vi "SetMotors (SubVI).vi"(6 "Oikea":dbl, 9 "Etu":dbl, 10 "Vasen":dbl, 11 "Taka":dbl) -> ()   [LabVIEW 2018]
uses:
  <vilib>/Utility/error.llb/Error Cluster From Error Code.vi
  <vilib>/myRIO/Common/Instrument Driver Framework/myRIO v1.0/PWM/vis/myRIO v1.0 Write PWM.vi
  <vilib>/myRIO/Instrument Drivers/Onboard IO/PWM/PWM.lvlib
panel:
  out "error out":errorcluster
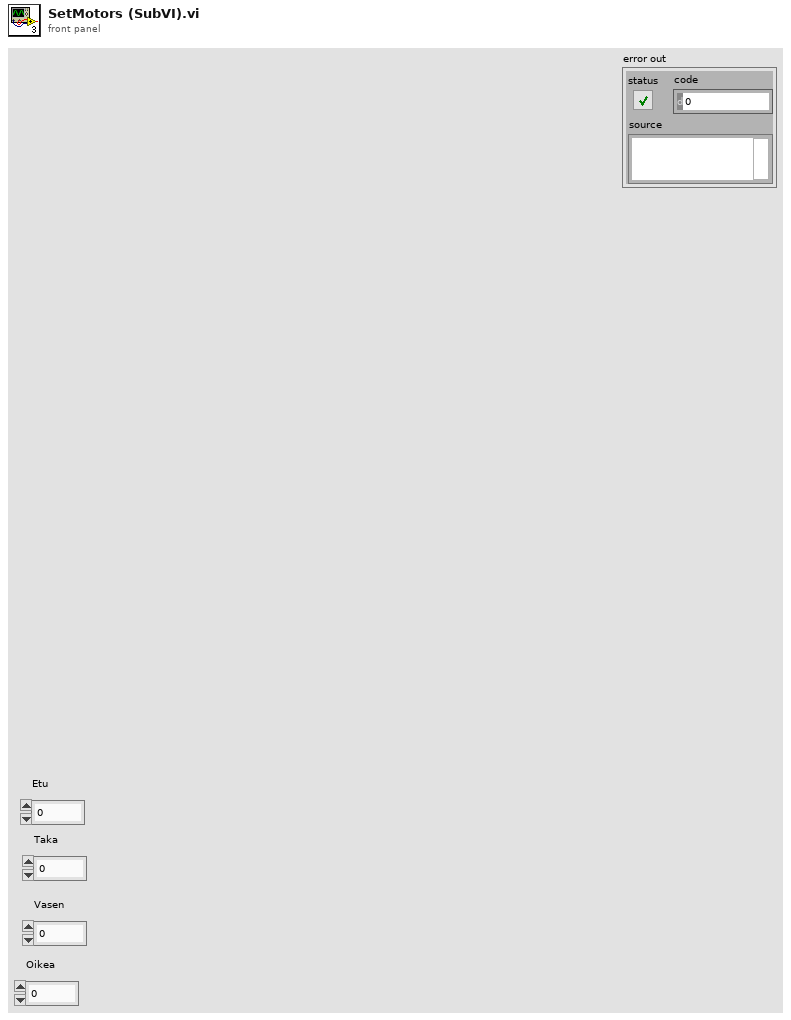
[diagram p1: front panel]
types:
  T1 = typedef "PWM.lvlib/PWM Reference.ctl" = cluster{"myRIO Reference":T2, "PWM Channels Enum":T6, "PWM Configuration":T7}
  T2 = typedef "myRIO Generic Hardware Reference.ctl" = cluster{"myRIO Model":T3, "myRIO Hardware Reference":T4}
  T3 = typedef "Hardware Version Enum.ctl" = enum16{"Unknown", "myRIO-1900", "myRIO-1950", "roboRIO", "NI ELVIS RIO CM", "ELVIS III"}
  T4 = typedef "myRIO v1.0 Reference.ctl" = cluster{"Generic FPGA Reference":T5, "Allow multiple opens":bool}
  T5 = typedef "Generic FPGA Reference.ctl" = refnum<k20>
  T6 = typedef "PWM Channels Enum.ctl" = enum16{"Not Connected", "C/PWM0", "C/PWM1", "A/PWM0", "A/PWM1", "A/PWM2", "A/PWM3", "A/PWM4", "A/PWM5", "A/PWM6", "A/PWM7", "A/PWM8", "A/PWM9", "A/PWM10", "A/PWM11", "A/PWM12", "A/PWM13", "A/PWM14", "A/PWM15", "A/PWM16", "A/PWM17", "A/PWM18", "A/PWM19", "B/PWM0", "B/PWM1", "B/PWM2", "B/PWM3", "B/PWM4", "B/PWM5", "B/PWM6", "B/PWM7", "B/PWM8", "B/PWM9", "B/PWM10", "B/PWM11", "B/PWM12", "B/PWM13", "B/PWM14", "B/PWM15", "B/PWM16", "B/PWM17", "B/PWM18", "B/PWM19", "PWM/PWM0", "PWM/PWM1", "PWM/PWM2", "PWM/PWM3", "PWM/PWM4", "PWM/PWM5", "PWM/PWM6", "PWM/PWM7", "PWM/PWM8", "PWM/PWM9"}
  T7 = typedef "PWM.lvlib/PWM Configuration.ctl" = cluster{"Frequency":dbl, "Duty Cycle":dbl}
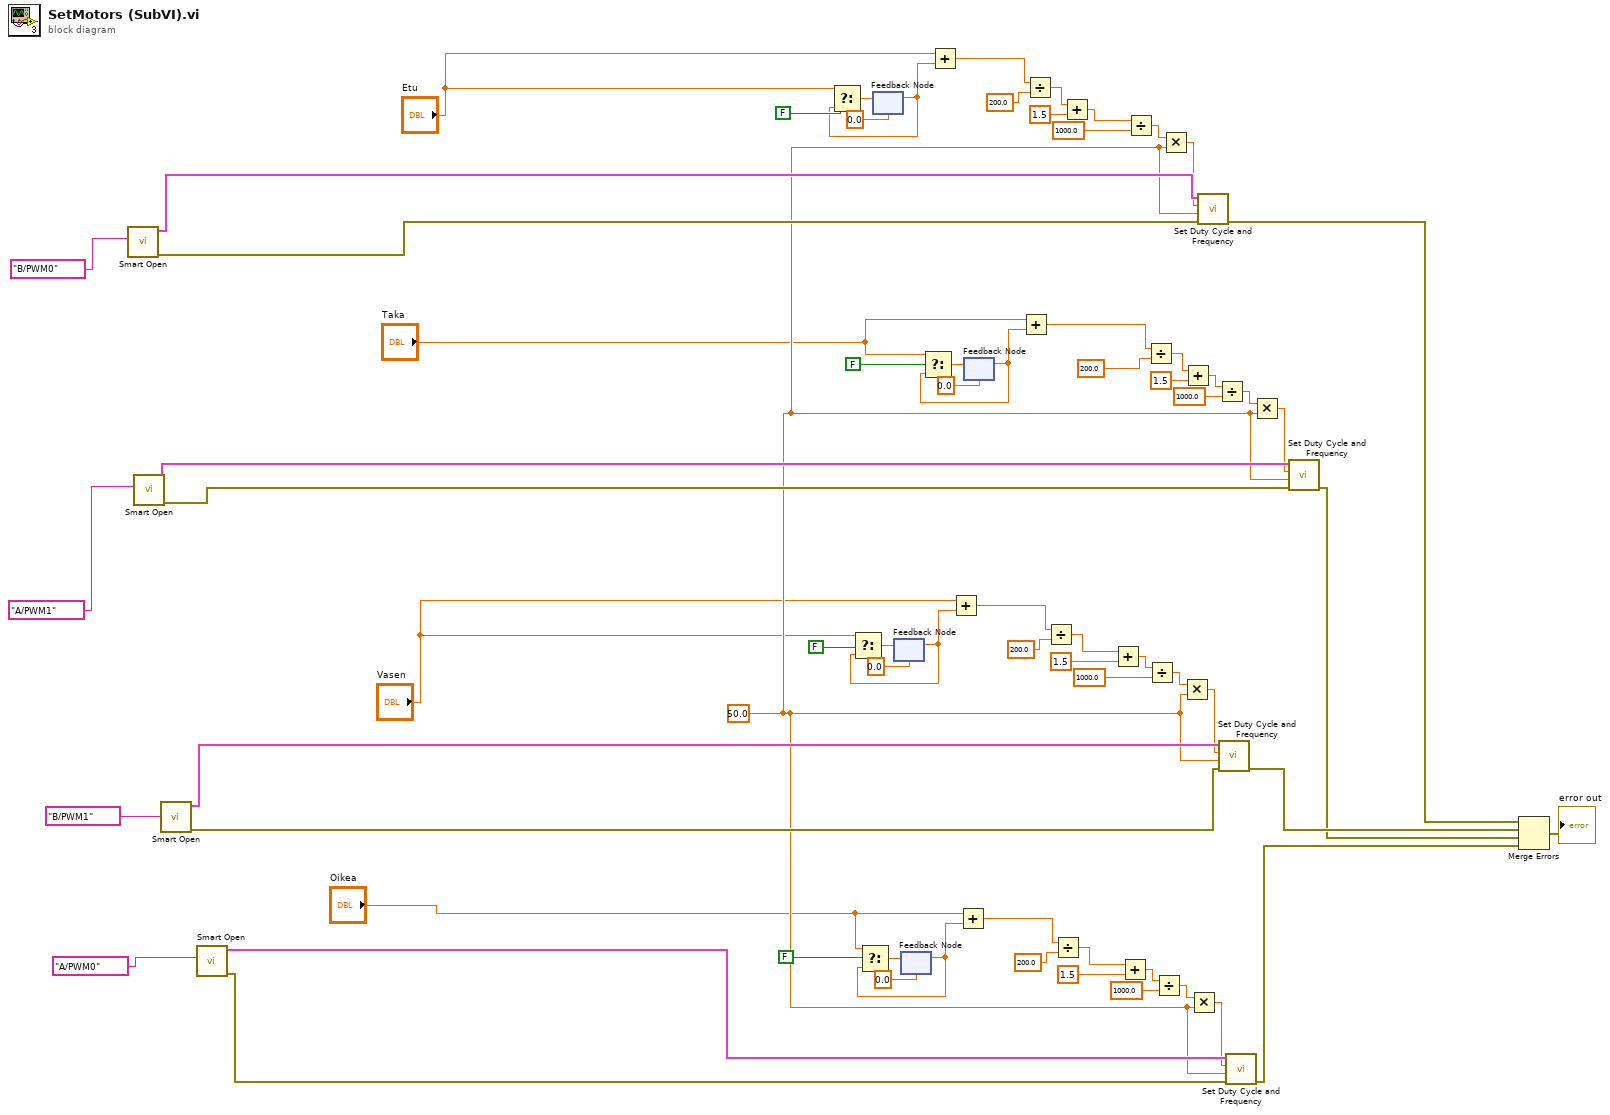
[diagram p0: block diagram]
diagram:
  w9 = 50.0 ("freq [Hz]")
  n1 = call <vilib>:"Smart Open.vi"("Channel Name"=tag "B/PWM0" ("PWM channel 4")) -> ("error out"=w60:errorcluster, "PWM Ref Out"=w61:T1)  [unwired: 9 in]
  n2 = call <vilib>:"Smart Open.vi"("Channel Name"=tag "A/PWM1" ("PWM channel 3")) -> ("error out"=w64:errorcluster, "PWM Ref Out"=w63:T1)  [unwired: 9 in]
  n3 = call <vilib>:"Smart Open.vi"("Channel Name"=tag "B/PWM1" ("PWM channel 2")) -> ("error out"=w59:errorcluster, "PWM Ref Out"=w66:T1)  [unwired: 9 in]
  n4 = call <vilib>:"Smart Open.vi"("Channel Name"=tag "A/PWM0" ("PWM channel")) -> ("error out"=w69:errorcluster, "PWM Ref Out"=w68:T1)  [unwired: 9 in]
  n5 = feedback #1(0.0 ("position [%FS]")) -> (w13:dbl)
  n6 = Select(t="Etu", s=FALSE ("null offset 6"), f=w13) -> (s? t:f=w15:dbl)
  n7 = feedback-in #1(w15) -> ()
  n8 = feedback #2(0.0 ("position [%FS]")) -> (w55:dbl)
  n9 = Select(t="Vasen", s=FALSE ("null offset 3"), f=w55) -> (s? t:f=w53:dbl)
  n10 = feedback-in #2(w53) -> ()
  n11 = feedback #3(0.0 ("position [%FS]")) -> (w38:dbl)
  n12 = Select(t="Oikea", s=FALSE ("null offset 4"), f=w38) -> (s? t:f=w40:dbl)
  n13 = feedback-in #3(w40) -> ()
  n14 = Add(x="Etu", y=w13) -> (x+y=w14:dbl)
  n15 = Add(x="Vasen", y=w55) -> (x+y=w54:dbl)
  n16 = Add(x="Oikea", y=w38) -> (x+y=w39:dbl)
  n17 = feedback #4(0.0 ("position [%FS]")) -> (w25:dbl)
  n18 = Select(t="Taka", s=FALSE ("null offset 5"), f=w25) -> (s? t:f=w27:dbl)
  n19 = feedback-in #4(w27) -> ()
  n20 = Add(x="Taka", y=w25) -> (x+y=w26:dbl)
  n21 = Divide(x=w14, y=200.0) -> (x/y=w20:dbl)
  n22 = Divide(x=w54, y=200.0) -> (x/y=w48:dbl)
  n23 = Divide(x=w39, y=200.0) -> (x/y=w45:dbl)
  n24 = Add(x=w20, y=1.5) -> (x+y=w18:dbl)
  n25 = Add(x=w48, y=1.5) -> (x+y=w50:dbl)
  n26 = Add(x=w45, y=1.5) -> (x+y=w43:dbl)
  n27 = Divide(x=w18, y=1000.0) -> (x/y=w12:dbl)
  n28 = Divide(x=w26, y=200.0) -> (x/y=w32:dbl)
  n29 = Divide(x=w50, y=1000.0) -> (x/y=w56:dbl)
  n30 = Divide(x=w43, y=1000.0) -> (x/y=w37:dbl)
  n31 = Multiply(x=w12, y=w9) -> (x*y=w11:dbl)
  n32 = Multiply(x=w56, y=w9) -> (x*y=w57:dbl)
  n33 = Add(x=w32, y=1.5) -> (x+y=w30:dbl)
  n34 = Multiply(x=w37, y=w9) -> (x*y=w36:dbl)
  n35 = call <vilib>:"Set Duty Cycle and Frequency.vi"("error in (no error)"=w60, "Frequency [Hz]"=w9, "Duty Cycle"=w11, "PWM Ref In"=w61) -> ("error out"=w8:errorcluster)  [unwired: 5 in, 1 out]
  n36 = Divide(x=w30, y=1000.0) -> (x/y=w24:dbl)
  n37 = call <vilib>:"Set Duty Cycle and Frequency.vi"("error in (no error)"=w59, "Frequency [Hz]"=w9, "Duty Cycle"=w57, "PWM Ref In"=w66) -> ("error out"=w3:errorcluster)  [unwired: 5 in, 1 out]
  n38 = call <vilib>:"Set Duty Cycle and Frequency.vi"("error in (no error)"=w69, "Frequency [Hz]"=w9, "Duty Cycle"=w36, "PWM Ref In"=w68) -> ("error out"=w1:errorcluster)  [unwired: 5 in, 1 out]
  n39 = Multiply(x=w24, y=w9) -> (x*y=w23:dbl)
  n40 = call <vilib>:"Set Duty Cycle and Frequency.vi"("error in (no error)"=w64, "Frequency [Hz]"=w9, "Duty Cycle"=w23, "PWM Ref In"=w63) -> ("error out"=w2:errorcluster)  [unwired: 5 in, 1 out]
  n41 = Merge Errors(w8, w3, w2, w1) -> (→"error out":errorcluster)
